vi "found pxi slot.vi"() -> ()   [LabVIEW 2015]
uses:
  <vilib>/Utility/error.llb/DialogType.ctl
  <vilib>/nisyscfg/Close (Hardware).vi
  <vilib>/nisyscfg/Close (System).vi
  <vilib>/nisyscfg/nisyscfg.lvlib
  <resource>/objmgr/nisysapi.rc
  <resource>/objmgr/nicriosae.rc
panel:
  out "Devices & Chassis:Product Name":string
  out "Devices & Chassis:Model Name Number":u32
  in  "stop":bool
  in  "error in (no error)":errorcluster
  out "error out":errorcluster
  in  "Target":refnum<k21>="NI-PXIe8135-2F217AF0 (192.168.150.78)"
  out "Devices & Chassis:Number Of Slots":i32
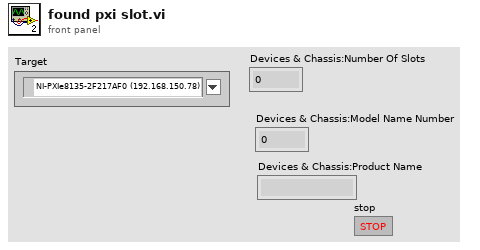
[diagram p1: front panel]
types:
  T1 = typedef "DialogType.ctl" = u16
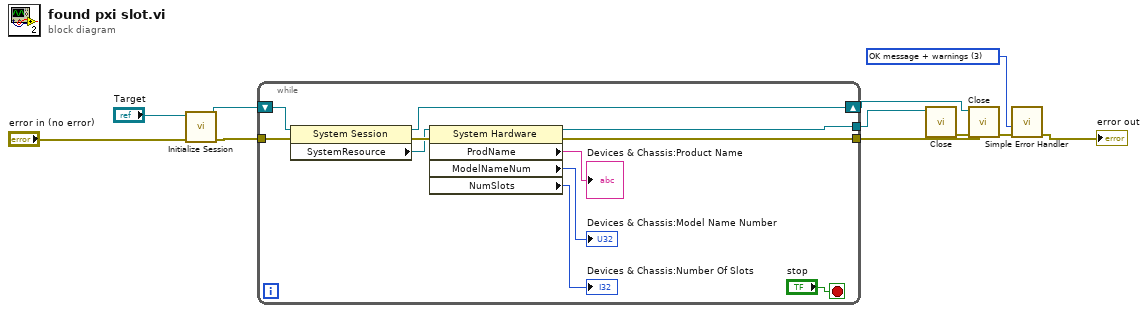
[diagram p0: block diagram]
diagram:
  w1 = T1 3 items=["no dialog", "OK message", "continue or stop message", "OK message + warnings", "continue/stop + warnings"] ("type of dialog (OK msg:1)")
  n1 = call <vilib>:"Initialize Session.vi"("error in (no error)"="error in (no error)", "Target (localhost)"="Target") -> ("error out"=w5:errorcluster, "Session out"=w6:refnum<k21>)  [unwired: 8 in]
  n2 = while {
    shift-right: [w18] -> w3
    shift-left: w6 -> [w20]
    tunnel: w5 -> [w19]
    tunnel: [w17] -> w4
    tunnel: [w16] -> w2
    stop <- "stop" stop-if-true
    n3 = property class="System Session"(reference=w20, error in=w19) -> (reference out=w18:refnum<k21>, error out=w22:errorcluster, "SystemResource"=w21:refnum<k20>)
    n4 = property class="System Hardware"(reference=w21, error in=w22) -> (reference out=w16:refnum<k20>, error out=w17:errorcluster, "ProdName"=→"Devices & Chassis:Product Name":string, "ModelNameNum"=→"Devices & Chassis:Model Name Number":u32, "NumSlots"=→"Devices & Chassis:Number Of Slots":i32)
  }
  n5 = call-poly <vilib>:"Close.vi"("error in (no error)"=w4, "Resource in"=w2) -> ("error out"=w10:errorcluster)  [unwired: 9 in]
  n6 = call-poly <vilib>:"Close.vi"("error in (no error)"=w10, "Session in"=w3) -> ("error out"=w11:errorcluster)  [unwired: 9 in]
  n7 = call <vilib>:"Simple Error Handler.vi"("type of dialog (OK msg:1)"=w1, "error in (no error)"=w11) -> ("error out"=→"error out":errorcluster)  [unwired: 3 in, 4 out]
